vi "Read GObj Ref.vi"(8 "error in (no error)":errorcluster, 11 "GObjectConverterBase in":refnum<class "GObjectConverterBase.lvclass">) -> (0 "error out":errorcluster, 2 "GObj Ref":refnum<vi>, 3 "GObjectConverterBase out":refnum<class "GObjectConverterBase.lvclass">)   [LabVIEW 2017, in "GObjectConverterBase.lvclass"]
uses:
  GObjectConverterBase.lvclass
  GObjectConverterBase.lvclass/GObjectConverterBase.ctl
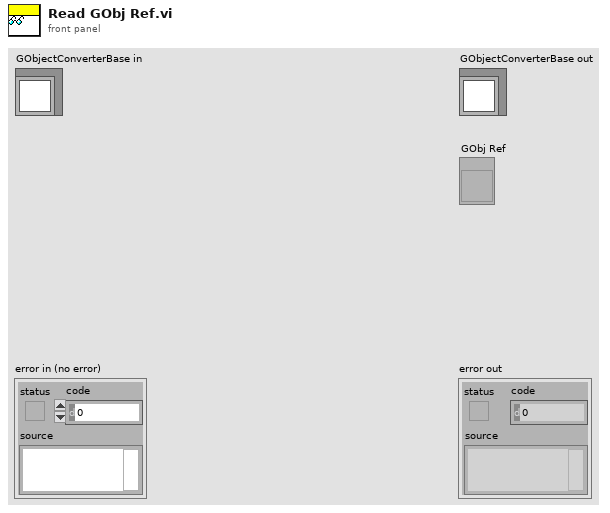
[diagram p1: front panel]
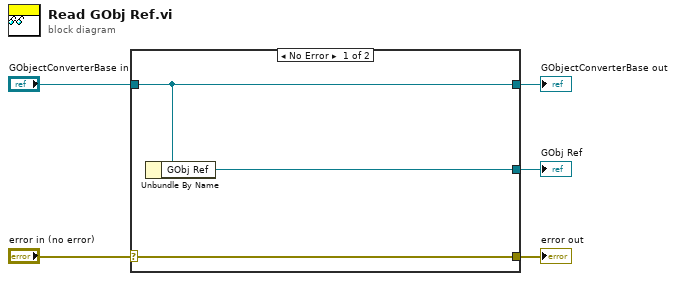
[diagram p0: block diagram]
diagram:
  n1 = case shown="No Error" "error in (no error)" {
    selector: "error in (no error)" -> [w8 w9]
    tunnel: [w8 w9] -> w4
    tunnel: [w7 w10] -> w2
    tunnel: "GObjectConverterBase in" -> [w7 w10]
    tunnel: [w6 _] -> w1
    frame No Error {
      n2 = Unbundle By Name(w7) -> ("GObj Ref"=w6:refnum<vi>)
    }
    frame Error {
    }
  }
  "error out" <- w4
  "GObjectConverterBase out" <- w2
  "GObj Ref" <- w1
